vi "KFold Indices.vi"(8 "error in (no error)":errorcluster, 9 "seed":i32=-1 caption="seed (-1)", 10 "Data size":i32=-1, 11 "Nr Folds":i32=5 caption="Nr Folds (5)") -> (0 "error out":errorcluster, 3 "Fold indices":cluster{i32[]}[](array[cluster]))   [LabVIEW 2015]
uses:
  <vilib>/Analysis/1siggen.llb/Riffle Array (I32).vi
  <vilib>/Analysis/NI_AALBase.lvlib
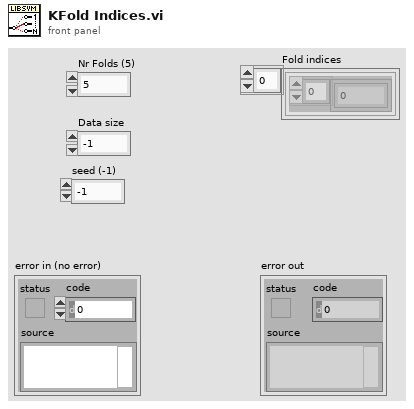
[diagram p1: front panel]
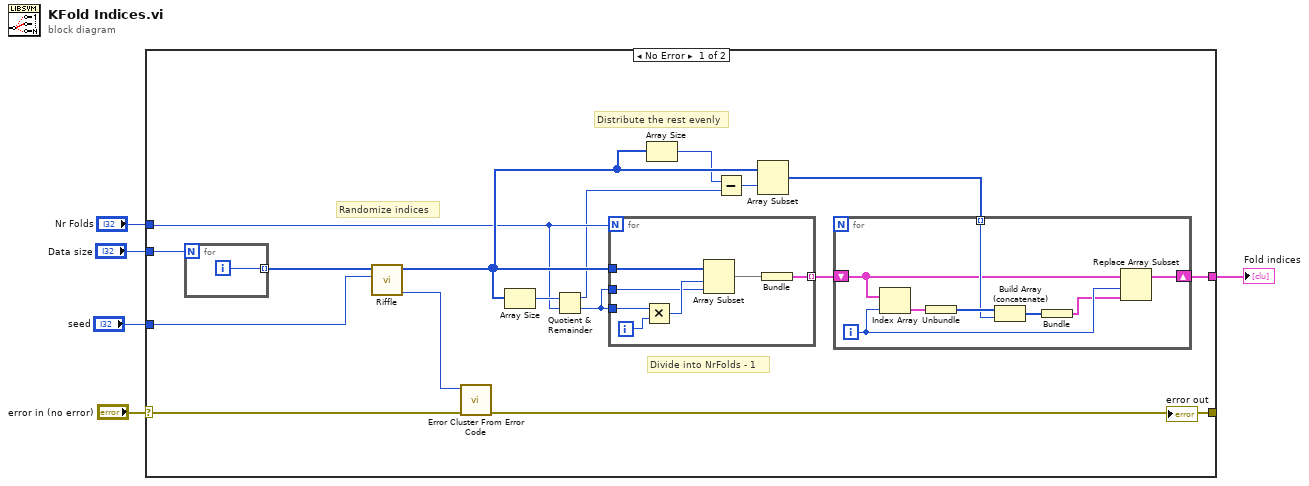
[diagram p0: block diagram]
diagram:
  n1 = case shown="No Error" "error in (no error)" {
    selector: "error in (no error)" -> [w19 w39]
    tunnel: [w18 w39] -> w6
    tunnel: "Data size" -> [w22 _]
    tunnel: "Nr Folds" -> [w9 _]
    tunnel: "seed" -> [w20 _]
    tunnel: [w10 _] -> w1
    frame No Error {
      # "Distribute the rest evenly"
      # "Randomize indices"
      # "Divide into NrFolds - 1"
      n2 = for {
        N: w22 -> [_]
        tunnel: [w38] -> w21 mode=indexing
        i -> [w38]
      }
      n3 = call-poly <vilib>:"Riffle.vi"("seed"=w20, "X"=w21) -> ("error"=w17:i32, "Riffled {X}"=w14:i32[])  [unwired: 7 in, 1 out]
      n4 = call <vilib>:"Error Cluster From Error Code.vi"("error in (no error)"=w19, "error code (0)"=w17) -> ("error out"=w18:errorcluster)  [unwired: 7 in]
      n5 = Array Size(array=w14) -> (size(s)=w15:i32)
      n6 = Quotient & Remainder(x=w15, y=w9) -> (x-y*floor(x/y)=w8:i32, floor(x/y)=w16:i32)
      n7 = for {
        N: w9 -> [_]
        tunnel: w14 -> [w37]
        tunnel: w16 -> [w36]
        tunnel: w16 -> [w33]
        tunnel: [w31] -> w12 mode=indexing
        i -> [w35]
        n8 = Multiply(x=w36, y=w35) -> (x*y=w34:i32)
        n9 = Array Subset(array=w37, index=w34, length=w33) -> (w32:i32[])
        n10 = Bundle(w32) -> (w31:cluster{i32[]})  [unwired: 1 in]
      }
      n11 = Array Size(array=w14) -> (size(s)=w7:i32)
      n12 = Subtract(x=w7, y=w8) -> (x-y=w13:i32)
      n13 = Array Subset(array=w14, index=w13) -> (w11:i32[])  [unwired: 1 in]
      n14 = for {
        tunnel: w11 -> [w28] mode=indexing
        shift-right: [w25] -> w10
        shift-left: w12 -> [w26]
        i -> [w24]
        n15 = Index Array(array=w26, index=w24) -> (element=w30:cluster{i32[]})
        n16 = Unbundle(w30) -> (w29:i32[])
        n17 = Build Array (concatenate)(w29, w28) -> (w27:i32[])
        n18 = Bundle(w27) -> (w23:cluster{i32[]})  [unwired: 1 in]
        n19 = Replace Array Subset(array=w26, new element=w23, index=w24) -> (w25:cluster{i32[]}[])
      }
    }
    frame Error {
    }
  }
  "error out" <- w6
  "Fold indices" <- w1
